vi "Get Desired Size.vi"(8 "error in (no error)":errorcluster, 11 "Value Editor Base in":refnum<class "Value Editor Base.lvclass">) -> (0 "error out":errorcluster, 2 "Desired Size":T1, 3 "Value Editor Base out":refnum<class "Value Editor Base.lvclass">)   [LabVIEW 2020, in "Value Editor Base.lvclass"]
uses:
  Value Editor Base.lvclass
  <vilib>/IlluminatedG/IG OOPanel/OOPanel/ArrayPanel/Desired Size.ctl
  Value Editor Base.lvclass/Value Editor Base.ctl
  <vilib>/IlluminatedG/IG OOPanel/OOPanel/OOPanel.lvlib
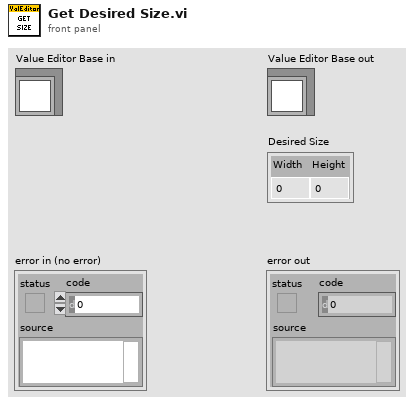
[diagram p1: front panel]
types:
  T1 = typedef "OOPanel.lvlib/Desired Size.ctl" = cluster{"Width":u32, "Height":u32}
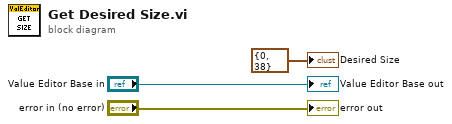
[diagram p0: block diagram]
diagram:
  "error out" <- "error in (no error)"
  "Value Editor Base out" <- "Value Editor Base in"
  "Desired Size" <- T1 {"Width"=0, "Height"=38} ("Desired Size")
